vi "Get Raw Data.vi"(8 "Error In":errorcluster, 9 "Number of Samples/ch (-1:all)":i32, 10 "Offset":i32, 11 "Path In":path) -> (0 "Error Out":errorcluster, 1 "T":dbl[](array[numeric]), 2 "Trace":T1(array[cluster]), 3 "Path Out":path)   [LabVIEW 2017, in "Aquisicao de Dados.lvlib"]
uses:
  Aquisicao de Dados.lvlib
  <vilib>/Utility/error.llb/whitespace.ctl
  <vilib>/gmath/NI_Gmath.lvlib
panel:
  out "Waveform Graph":dbl[](graph)
  out "data":string
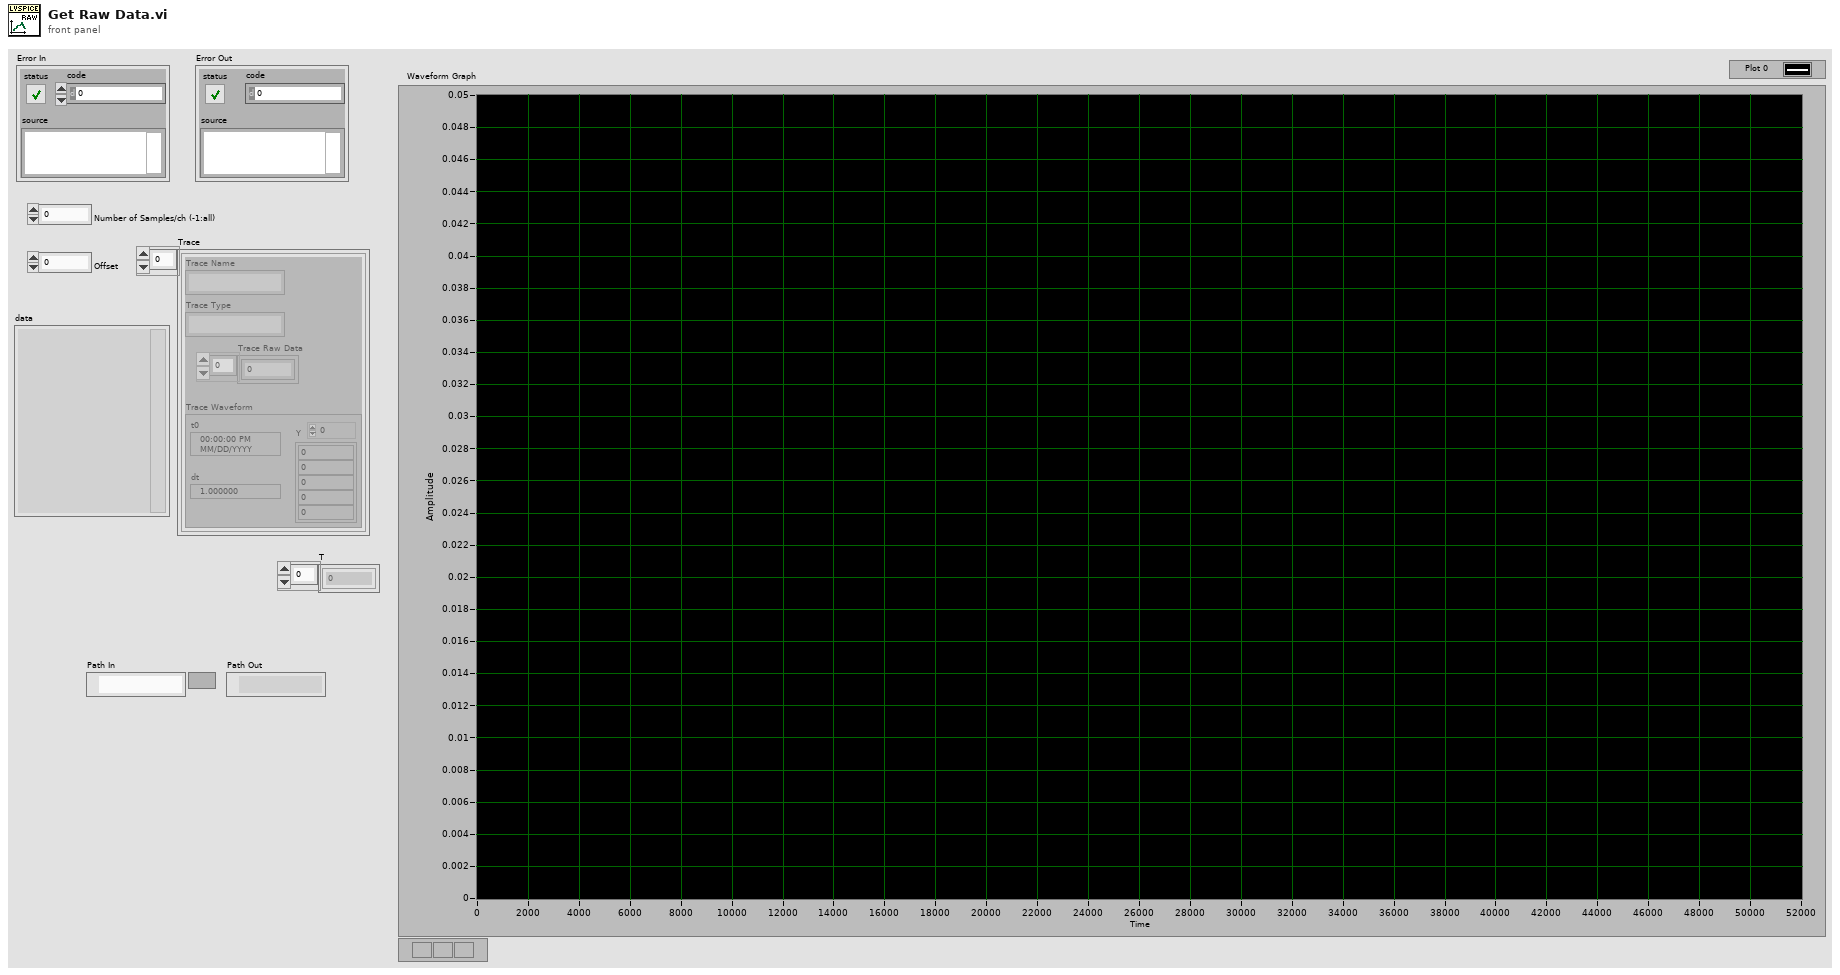
[diagram p1: front panel]
types:
  T1 = cluster{"Trace Name":string, "Trace Type":string, "Trace Raw Data":dbl[], "Trace Waveform":waveform(dbl)}[]
  T2 = cluster{"Field Name":string, "Field Data":variant}
  T3 = typedef "whitespace.ctl" = u16
  T4 = cluster{"Trace Name":string, "Trace Type":string, "Trace Raw Data":dbl[], "Trace Waveform":waveform(dbl)}
  T5 = cluster{"Field Name":string, "Field Data":variant}[]
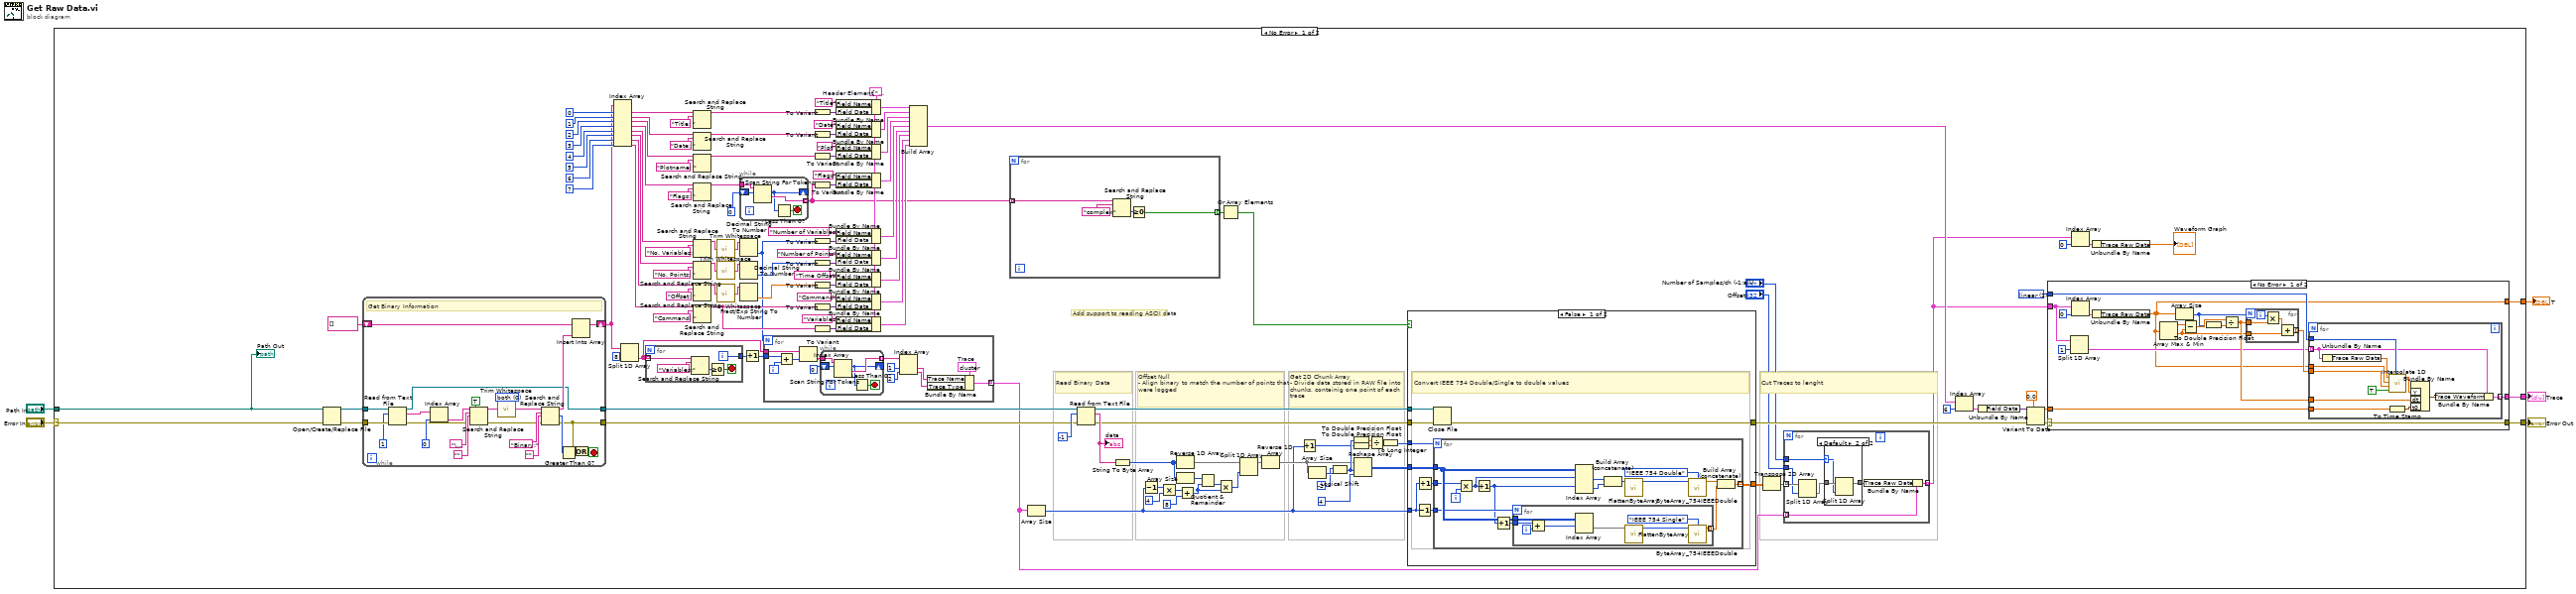
[diagram p0: block diagram]
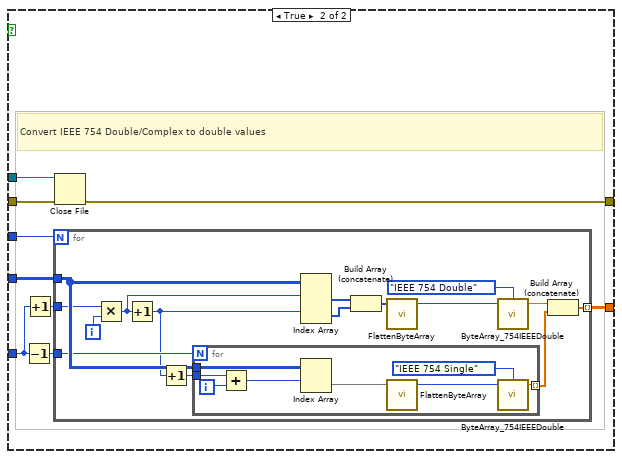
[diagram p2: hidden frame]
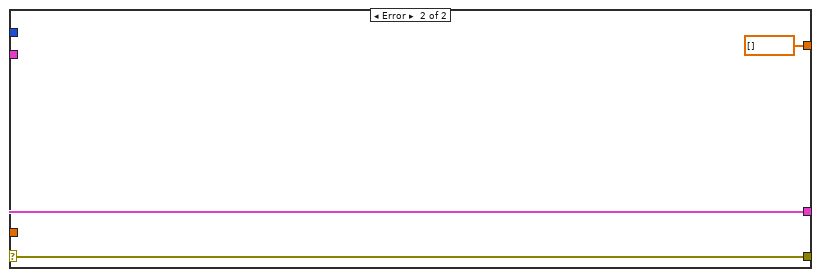
[diagram p3: hidden frame]
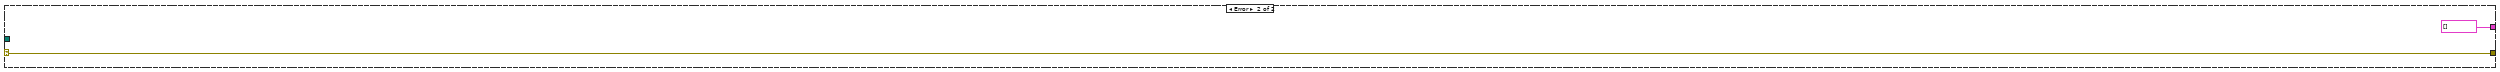
[diagram p5: hidden frame]
diagram:
  n1 = case shown="No Error" "Error In" {
    selector: "Error In" -> [w133 w304]
    tunnel: [w135 w304] -> w4
    tunnel: [w134 T1 []] -> w3
    tunnel: [w132 _] -> w2
    tunnel: "Path In" -> [w6 _]
    frame No Error {
      w39 = T2 {"Field Name"="", "Field Data"=variant}  # Header Element
      w95 = 1 items=["nearest", "linear", "spline", "cubic Hermite", "Lagrange"] ("method")
      # "Get 2D Chunk Array\n- Divide data stored in RAW file into chunks, containig one point of each trace"
      # "Add support to reading ASCII data"
      # "Offset Null\n- Align binary to match the number of points that were logged"
      # "Read Binary Data"
      # "Cut Traces to lenght"
      n2 = Open/Create/Replace File(file path (use dialog)=w6, error in=w133) -> (refnum out=w17:refnum<file>, error out=w18:errorcluster)  [unwired: 4 in, 1 out]
      n3 = while {
        tunnel: w17 -> [w254]
        tunnel: w18 -> [w253]
        shift-right: [w239] -> w23
        shift-left: string[] [] -> [w238]
        tunnel: [w233] -> w103
        tunnel: [w235] -> w104
        stop <- w232 stop-if-true
        w247 = T3 0 items=["both", "start of string", "end of string"] ("location (both)")
        # "Get Binary Information"
        n4 = Read from Text File(file (use dialog)=w254, count=1, error in=w253) -> (refnum out=w235:refnum<file>, text=w251:string[], error out=w237:errorcluster)  [unwired: 1 in, 1 out]
        n5 = Index Array(array=w251, index=0) -> (element=w245:string)
        n6 = Search and Replace String(replace all?=TRUE ("replace all? (F)"), input string=w245, search string="\u0000", replace string="" ("replace string (\"\")"), error in=w237) -> (result string=w243:string, error out=w236:errorcluster)  [unwired: 3 in, 2 out]
        n7 = call <vilib>:"Trim Whitespace.vi"("string"=w243, "location (both)"=w247) -> ("trimmed string"=w240:string)
        n8 = Search and Replace String(input string=w240, search string="Binary:", replace string="" ("replace string (\"\")"), error in=w236) -> (number of replacements=w248:i32, error out=w233:errorcluster)  [unwired: 4 in, 2 out]
        n9 = Greater Than 0?(x=w248) -> (x > 0?=w234:bool)
        n10 = Insert Into Array(array=w238, new element=w240) -> (w239:string[])  [unwired: 1 in]
        n11 = Or(x=w233, y=w234) -> (x .or. y?=w232:bool)
      }
      n12 = Index Array(array=w23, index #1=0 ("index"), index #2=1 ("index"), index #3=2 ("index"), index #4=3 ("index"), index #5=4 ("index"), index #6=5 ("index"), index #7=6 ("index"), index #8=7 ("index")) -> (element #1=w71:string, element #2=w70:string, element #3=w69:string, element #4=w68:string, element #5=w67:string, element #6=w66:string, element #7=w65:string, element #8=w64:string)
      n13 = Split 1D Array(array=w23, index=8) -> (second subarray=w21:string[])  [unwired: 1 out]
      n14 = for {
        tunnel: w21 -> [w225] mode=indexing
        tunnel: [w224] -> w20
        i -> [w224]
        stop <- w222 stop-if-true
        n15 = Search and Replace String(input string=w225, search string="Variables:" ("search string/char (-)")) -> (offset past replacement=w223:i32)  [unwired: 6 in, 3 out]
        n16 = Greater Or Equal To 0?(x=w223) -> (x >= 0?=w222:bool)
      }
      n17 = Search and Replace String(input string=w71, search string="Title: " ("search string/char (-)")) -> (result string=w38:string)  [unwired: 6 in, 3 out]
      n18 = Search and Replace String(input string=w70, search string="Date: " ("search string/char (-)")) -> (result string=w37:string)  [unwired: 6 in, 3 out]
      n19 = Search and Replace String(input string=w69, search string="Plotname: " ("search string/char (-)")) -> (result string=w36:string)  [unwired: 6 in, 3 out]
      n20 = Search and Replace String(input string=w68, search string="Flags: " ("search string/char (-)")) -> (result string=w29:string)  [unwired: 6 in, 3 out]
      n21 = Search and Replace String(input string=w67, search string="No. Variables: " ("search string/char (-)")) -> (result string=w30:string)  [unwired: 6 in, 3 out]
      n22 = Search and Replace String(input string=w66, search string="No. Points: " ("search string/char (-)")) -> (result string=w34:string)  [unwired: 6 in, 3 out]
      n23 = Search and Replace String(input string=w65, search string="Offset: " ("search string/char (-)")) -> (result string=w27:string)  [unwired: 6 in, 3 out]
      n24 = Search and Replace String(input string=w64, search string="Command: " ("search string/char (-)")) -> (result string=w35:string)  [unwired: 6 in, 3 out]
      n25 = call <vilib>:"Trim Whitespace.vi"("string"=w30) -> ("trimmed string"=w31:string)  [unwired: 1 in]
      n26 = call <vilib>:"Trim Whitespace.vi"("string"=w34) -> ("trimmed string"=w33:string)  [unwired: 1 in]
      n27 = call <vilib>:"Trim Whitespace.vi"("string"=w27) -> ("trimmed string"=w28:string)  [unwired: 1 in]
      n28 = while {
        tunnel: [w229] -> w9 mode=indexing
        tunnel: w29 -> [w230]
        shift-right: [w228] -> _
        shift-left: 0 ("offset past token") -> [w227]
        stop <- w231 stop-if-true
        n29 = Scan String For Tokens(8:w227, 9:w230) -> (1:w229:string, 2:w228:i32)  [unwired: 4 in, 2 out]
        n30 = Less Than 0?(x=w228) -> (x < 0?=w231:bool)
      }
      n31 = Decimal String To Number(string=w31) -> (number=w24:i32)  [unwired: 2 in, 1 out]
      n32 = Decimal String To Number(string=w33) -> (number=w32:i32)  [unwired: 2 in, 1 out]
      n33 = Fract/Exp String To Number(string=w28) -> (number=w26:dbl)  [unwired: 3 in, 1 out]
      n34 = Increment(x=w20) -> (x+1=w19:i32)
      n35 = for {
        N: w24 -> [_]
        tunnel: w19 -> [w215]
        tunnel: w21 -> [w216]
        tunnel: [w204] -> w102 mode=indexing
        i -> [w214]
        w207 = T4 {"Trace Name"="", "Trace Type"="", "Trace Raw Data"=[], "Trace Waveform"={"t0"=timestamp(0 s since 1904-01-01), "dt"=1.0, "Y"=[]}}  # Trace
        n36 = Add(x=w215, y=w214) -> (x+y=w213:i32)
        n37 = Index Array(array=w216, index=w213) -> (element=w211:string)
        n38 = while {
          tunnel: [w219] -> w210 mode=indexing
          tunnel: w211 -> [w220]
          shift-right: [w218] -> _
          shift-left: 0 ("offset past token") -> [w217]
          stop <- w221 stop-if-true
          n39 = Scan String For Tokens(8:w217, 9:w220) -> (1:w219:string, 2:w218:i32)  [unwired: 4 in, 2 out]
          n40 = Less Than 0?(x=w218) -> (x < 0?=w221:bool)
        }
        n41 = Index Array(array=w210, index #1=1 ("index"), index #2=2 ("index")) -> (element #1=w209:string, element #2=w208:string)
        n42 = Bundle By Name(cluster=w207, "Trace Name"=w209, "Trace Type"=w208) -> (w204:T4)
      }
      n43 = To Variant(anything=w38) -> (Variant=w87:variant)
      n44 = To Variant(anything=w37) -> (Variant=w63:variant)
      n45 = To Variant(anything=w36) -> (Variant=w59:variant)
      n46 = To Variant(anything=w9) -> (Variant=w58:variant)
      n47 = To Variant(anything=w24) -> (Variant=w55:variant)
      n48 = To Variant(anything=w32) -> (Variant=w54:variant)
      n49 = To Variant(anything=w26) -> (Variant=w51:variant)
      n50 = To Variant(anything=w35) -> (Variant=w50:variant)
      n51 = To Variant(anything=w35) -> (Variant=w47:variant)
      n52 = Bundle By Name(cluster=w39, "Field Name"="Title", "Field Data"=w87) -> (w61:T2)
      n53 = Bundle By Name(cluster=w39, "Field Name"="Date", "Field Data"=w63) -> (w46:T2)
      n54 = Bundle By Name(cluster=w39, "Field Name"="Plot", "Field Data"=w59) -> (w45:T2)
      n55 = Bundle By Name(cluster=w39, "Field Name"="Flags", "Field Data"=w58) -> (w10:T2)
      n56 = Bundle By Name(cluster=w39, "Field Name"="Number of Variables", "Field Data"=w55) -> (w44:T2)
      n57 = Bundle By Name(cluster=w39, "Field Name"="Number of Points", "Field Data"=w54) -> (w43:T2)
      n58 = Bundle By Name(cluster=w39, "Field Name"="Time Offset", "Field Data"=w51) -> (w42:T2)
      n59 = Bundle By Name(cluster=w39, "Field Name"="Command", "Field Data"=w50) -> (w41:T2)
      n60 = Bundle By Name(cluster=w39, "Field Name"="Variables", "Field Data"=w47) -> (w40:T2)
      n61 = Build Array(w61, w46, w45, w10, w44, w43, w42, w41, w40) -> (w94:T5)
      n62 = for {
        tunnel: w9 -> [w202] mode=indexing
        tunnel: [w200] -> w8 mode=indexing
        n63 = Search and Replace String(input string=w202, search string="complex" ("search string/char (-)")) -> (offset past replacement=w201:i32)  [unwired: 6 in, 3 out]
        n64 = Greater Or Equal To 0?(x=w201) -> (x >= 0?=w200:bool)
      }
      n65 = Array Size(array=w102) -> (size(s)=w12:i32)
      n66 = Read from Text File(file (use dialog)=w104, count=-1 ("count (1)"), error in=w103) -> (refnum out=w105:refnum<file>, text=w125:string, error out=w123:errorcluster)  [unwired: 1 in, 1 out]
      "data" <- w125
      n67 = String To Byte Array(string=w125) -> (unsigned byte array=w126:u8[])
      n68 = Decrement(x=w12) -> (x-1=w122:i32)
      n69 = Multiply(x=w122, y=4) -> (x*y=w112:i32)
      n70 = Reverse 1D Array(array=w126) -> (reversed array=w128:u8[])
      n71 = Array Size(array=w126) -> (size(s)=w127:i32)
      n72 = Add(x=w112, y=8 ("x")) -> (x+y=w120:i32)
      n73 = Quotient & Remainder(x=w127, y=w120) -> (floor(x/y)=w131:i32)  [unwired: 1 out]
      n74 = Multiply(x=w131, y=w120) -> (x*y=w129:i32)
      n75 = Or Array Elements(Boolean array=w8) -> (logical OR=w7:bool)
      n76 = Split 1D Array(array=w128, index=w129) -> (first subarray=w130:u8[])  [unwired: 1 out]
      n77 = Reverse 1D Array(array=w130) -> (reversed array=w113:u8[])
      n78 = Increment(x=w12) -> (x+1=w11:i32)
      n79 = Array Size(array=w113) -> (size(s)=w118:i32)
      n80 = Logical Shift(y=i16 -2, x=w118) -> (x << y=w115:i32)
      n81 = To Double Precision Float(number=w115) -> (double precision float=w114:dbl)
      n82 = To Double Precision Float(number=w11) -> (double precision float=w110:dbl)
      n83 = Reshape Array(w113, w115, 4 ("dimension size")) -> (w109:u8[][])
      n84 = Divide(x=w114, y=w110) -> (x/y=w116:dbl)
      n85 = To Long Integer(number=w116) -> (32bit integer=w108:i32)
      n86 = case shown="False" w7 {
        tunnel: w123 -> [w144 w176]
        tunnel: w109 -> [w143 w175]
        tunnel: w108 -> [w142 w174]
        tunnel: [w141 w173] -> w107
        tunnel: w105 -> [w138 w170]
        tunnel: [w137 w169] -> w93
        tunnel: w12 -> [w136 w168]
        frame False {
          # "Convert IEEE 754 Double/Single to double values"
          n87 = Decrement(x=w136) -> (x-1=w140:i32)
          n88 = Increment(x=w136) -> (x+1=w139:i32)
          n89 = for {
            N: w142 -> [_]
            tunnel: w143 -> [w153]
            tunnel: [w149] -> w141 mode=indexing
            tunnel: w140 -> [w148]
            tunnel: w139 -> [w147]
            i -> [w159]
            n90 = Multiply(x=w147, y=w159) -> (x*y=w158:i32)
            n91 = Increment(x=w158) -> (x+1=w145:i32)
            n92 = Increment(x=w145) -> (x+1=w152:i32)
            n93 = for {
              N: w148 -> [_]
              tunnel: w153 -> [w165]
              tunnel: w152 -> [w167]
              tunnel: [w162] -> w150 mode=indexing
              i -> [w166]
              n94 = Add(x=w167, y=w166) -> (x+y=w161:i32)
              n95 = Index Array(array=w165, index (row)=w161) -> (element=w160:u8[])  [unwired: 1 in]
              n96 = call "FlattenByteArray.vi"("Byte Array"=w160) -> ("QWord Out"=w164:u64)  [unwired: 3 in]
              n97 = call "ByteArray_754IEEEDouble.vi"("Byte Array In"=w164, "Output Format"=enum16{"IEEE 754 Single", "IEEE 754 Double"}."IEEE 754 Single") -> ("IEEE Double Out"=w162:dbl)  [unwired: 3 in]
            }
            n98 = Index Array(array=w153, index (row) #1=w158, index (row) #2=w145) -> (element #1=w157:u8[], element #2=w146:u8[])  [unwired: 2 in]
            n99 = Build Array (concatenate)(w157, w146) -> (w155:u8[])
            n100 = call "FlattenByteArray.vi"("Byte Array"=w155) -> ("QWord Out"=w154:u64)  [unwired: 3 in]
            n101 = call "ByteArray_754IEEEDouble.vi"("Byte Array In"=w154, "Output Format"=enum16{"IEEE 754 Single", "IEEE 754 Double"}."IEEE 754 Double") -> ("IEEE Double Out"=w151:dbl)  [unwired: 3 in]
            n102 = Build Array (concatenate)(w151, w150) -> (w149:dbl[])
          }
          n103 = Close File(refnum=w138, error in=w144) -> (error out=w137:errorcluster)  [unwired: 1 out]
        }
        frame True {
          # "Convert IEEE 754 Double/Complex to double values"
          n104 = Decrement(x=w168) -> (x-1=w172:i32)
          n105 = Increment(x=w168) -> (x+1=w171:i32)
          n106 = for {
            N: w174 -> [_]
            tunnel: w175 -> [w185]
            tunnel: [w181] -> w173 mode=indexing
            tunnel: w172 -> [w180]
            tunnel: w171 -> [w179]
            i -> [w191]
            n107 = Multiply(x=w179, y=w191) -> (x*y=w190:i32)
            n108 = Increment(x=w190) -> (x+1=w177:i32)
            n109 = Increment(x=w177) -> (x+1=w184:i32)
            n110 = for {
              N: w180 -> [_]
              tunnel: w185 -> [w197]
              tunnel: w184 -> [w199]
              tunnel: [w194] -> w182 mode=indexing
              i -> [w198]
              n111 = Add(x=w199, y=w198) -> (x+y=w193:i32)
              n112 = Index Array(array=w197, index (row)=w193) -> (element=w192:u8[])  [unwired: 1 in]
              n113 = call "FlattenByteArray.vi"("Byte Array"=w192) -> ("QWord Out"=w196:u64)  [unwired: 3 in]
              n114 = call "ByteArray_754IEEEDouble.vi"("Byte Array In"=w196, "Output Format"=enum16{"IEEE 754 Single", "IEEE 754 Double"}."IEEE 754 Single") -> ("IEEE Double Out"=w194:dbl)  [unwired: 3 in]
            }
            n115 = Index Array(array=w185, index (row) #1=w190, index (row) #2=w177) -> (element #1=w189:u8[], element #2=w178:u8[])  [unwired: 2 in]
            n116 = Build Array (concatenate)(w189, w178) -> (w187:u8[])
            n117 = call "FlattenByteArray.vi"("Byte Array"=w187) -> ("QWord Out"=w186:u64)  [unwired: 3 in]
            n118 = call "ByteArray_754IEEEDouble.vi"("Byte Array In"=w186, "Output Format"=enum16{"IEEE 754 Single", "IEEE 754 Double"}."IEEE 754 Double") -> ("IEEE Double Out"=w183:dbl)  [unwired: 3 in]
            n119 = Build Array (concatenate)(w183, w182) -> (w181:dbl[])
          }
          n120 = Close File(refnum=w170, error in=w176) -> (error out=w169:errorcluster)  [unwired: 1 out]
        }
      }
      n121 = Transpose 2D Array(2D array=w107) -> (transposed array=w106:dbl[][])
      n122 = for {
        tunnel: w102 -> [w298] mode=indexing
        tunnel: w106 -> [w296] mode=indexing
        tunnel: [w297] -> w14 mode=indexing
        tunnel: "Offset" -> [w294]
        tunnel: "Number of Samples/ch (-1:all)" -> [w292]
        n123 = Split 1D Array(array=w296, index=w294) -> (second subarray=w295:dbl[])  [unwired: 1 out]
        n124 = case shown="Default" w292 {
          selector: w292 -> [_ w300]
          tunnel: w295 -> [w299 w302]
          tunnel: [w299 w301] -> w293
          frame -1 {
          }
          frame Default {
            n125 = Split 1D Array(array=w302, index=w300) -> (first subarray=w301:dbl[])  [unwired: 1 out]
          }
        }
        n126 = Bundle By Name(cluster=w298, "Trace Raw Data"=w293) -> (w297:T4)
      }
      n127 = Index Array(array=w94, index=6) -> (element=w98:T2)
      n128 = Unbundle By Name(w98) -> ("Field Data"=w99:variant)
      n129 = Variant To Data(error in=w93, type=0.0 ("min value"), Variant=w99) -> (data=w96:dbl, error out=w97:errorcluster)
      n130 = case shown="No Error" w97 {
        selector: w97 -> [w256 w290]
        tunnel: w14 -> [w263 w291]
        tunnel: w96 -> [w259 _]
        tunnel: w95 -> [w258 _]
        tunnel: [w257 w291] -> w134
        tunnel: [w256 w290] -> w135
        tunnel: [w255 dbl[] [] ("Trace Raw Data")] -> w132
        frame No Error {
          n131 = Split 1D Array(array=w263, index=1) -> (second subarray=w260:T1)  [unwired: 1 out]
          n132 = Index Array(array=w263, index=0) -> (element=w261:T4)
          n133 = Unbundle By Name(w261) -> ("Trace Raw Data"=w255:dbl[])
          n134 = Array Max & Min(array=w255) -> (max value=w265:dbl, min value=w270:dbl)  [unwired: 2 out]
          n135 = Array Size(array=w255) -> (size(s)=w267:i32)
          n136 = Subtract(x=w265, y=w270) -> (x-y=w269:dbl)
          n137 = To Double Precision Float(number=w267) -> (double precision float=w266:dbl)
          n138 = Divide(x=w269, y=w266) -> (x/y=w271:dbl)
          n139 = for {
            N: w267 -> [_]
            tunnel: w270 -> [w286]
            tunnel: w271 -> [w287]
            tunnel: [w284] -> w268 mode=indexing
            i -> [w288]
            n140 = Multiply(x=w288, y=w287) -> (x*y=w285:dbl)
            n141 = Add(x=w285, y=w286) -> (x+y=w284:dbl)
          }
          n142 = for {
            tunnel: w271 -> [w283]
            tunnel: w268 -> [w280]
            tunnel: w255 -> [w278]
            tunnel: w260 -> [w274] mode=indexing
            tunnel: w258 -> [w276]
            tunnel: w259 -> [w275]
            tunnel: [w272] -> w257 mode=indexing
            n143 = Unbundle By Name(w274) -> ("Trace Raw Data"=w277:dbl[])
            n144 = call <vilib>:"Interpolate 1D.vi"("method"=w276, "X is monotonic"=TRUE, "xi"=w280, "X"=w278, "Y"=w277) -> ("yi"=w281:dbl[])  [unwired: 4 in, 2 out]
            n145 = To Time Stamp(1:w275) -> (0:w282:timestamp)
            n146 = Bundle By Name("Y"=w281, "dt"=w283, "t0"=w282) -> (w273:waveform(dbl))  [unwired: 1 in]
            n147 = Bundle By Name(cluster=w274, "Trace Waveform"=w273) -> (w272:T4)
          }
        }
        frame Error {
        }
      }
      n148 = Index Array(array=w14, index=0) -> (element=w16:T4)
      n149 = Unbundle By Name(w16) -> ("Trace Raw Data"=→"Waveform Graph":dbl[])
      "Path Out" <- w6
    }
    frame Error {
    }
  }
  "Error Out" <- w4
  "Trace" <- w3
  "T" <- w2
